vi "Convert To Child Class.vi"(11 "MetaDataObj in":refnum<class "MetaDataObj.lvclass">) -> (3 "MetaDataObj out":refnum<class "MetaDataObj.lvclass">)   [LabVIEW 2016, in "MetaDataObj.lvclass"]
uses:
  <resource>/dialog/NewProjectWizard/MetaDataObj/MetaDataObj.lvclass
  <resource>/dialog/NewProjectWizard/MetaDataObj/MetaDataObj.lvclass/MetaDataObj.ctl
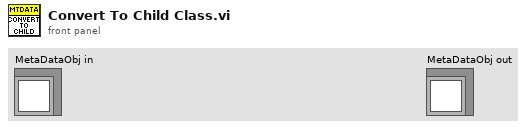
[diagram p1: front panel]
types:
  T1 = typedef "CustomVIModes.ctl" = enum16{"None", "AfterPage1", "AfterPage2WithUI", "AfterPage2NoUI"}
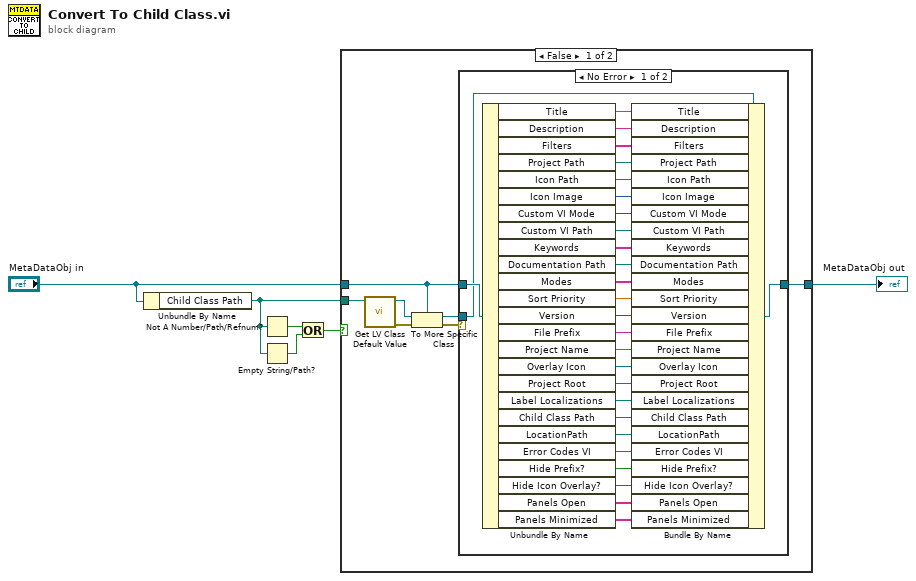
[diagram p0: block diagram]
diagram:
  n1 = Unbundle By Name("MetaDataObj in") -> ("Child Class Path"=w1:path)
  n2 = Not A Number/Path/Refnum?(number/path/refnum=w1) -> (NaN/Path/Refnum?=w6:bool)
  n3 = Empty String/Path?(string/path=w1) -> (empty?=w5:bool)
  n4 = Or(x=w6, y=w5) -> (x .or. y?=w4:bool)
  n5 = case shown="False" w4 {
    tunnel: [w8 w43] -> w3
    tunnel: "MetaDataObj in" -> [w9 w43]
    tunnel: w1 -> [w13 _]
    frame False {
      n6 = call <vilib>:"Get LV Class Default Value.vi"("class path"=w13) -> ("error out"=w7:errorcluster, "object"=w12:refnum<class>)  [unwired: 9 in]
      n7 = To More Specific Class(target class=w9, reference=w12, error in=w7) -> (specific class reference=w10:refnum<class "MetaDataObj.lvclass">, error out=w11:errorcluster)
      n8 = case shown="No Error" w11 {
        tunnel: w10 -> [w40 _]
        tunnel: w9 -> [w41 w42]
        tunnel: [w39 w42] -> w8
        frame No Error {
          n9 = Unbundle By Name(w41) -> ("Title"=w38:string, "Description"=w37:string, "Filters"=w36:string[], "Project Path"=w35:path, "Icon Path"=w34:path, "Icon Image"=w33:picture, "Custom VI Mode"=w32:T1, "Custom VI Path"=w31:path, "Keywords"=w30:string[], "Documentation Path"=w29:path, "Modes"=w28:string[], "Sort Priority"=w27:dbl, "Version"=w26:u8, "File Prefix"=w25:string, "Project Name"=w24:string, "Overlay Icon"=w23:refnum<class "Icon.lvclass">, "Project Root"=w22:path, "Label Localizations"=w21:path, "Child Class Path"=w20:path, "LocationPath"=w19:path, "Error Codes VI"=w18:path, "Hide Prefix?"=w17:bool, "Hide Icon Overlay?"=w16:bool, "Panels Open"=w15:string[], "Panels Minimized"=w14:string[])
          n10 = Bundle By Name(cluster=w40, "Title"=w38, "Description"=w37, "Filters"=w36, "Project Path"=w35, "Icon Path"=w34, "Icon Image"=w33, "Custom VI Mode"=w32, "Custom VI Path"=w31, "Keywords"=w30, "Documentation Path"=w29, "Modes"=w28, "Sort Priority"=w27, "Version"=w26, "File Prefix"=w25, "Project Name"=w24, "Overlay Icon"=w23, "Project Root"=w22, "Label Localizations"=w21, "Child Class Path"=w20, "LocationPath"=w19, "Error Codes VI"=w18, "Hide Prefix?"=w17, "Hide Icon Overlay?"=w16, "Panels Open"=w15, "Panels Minimized"=w14) -> (w39:refnum<class "MetaDataObj.lvclass">)
        }
        frame Error {
        }
      }
    }
    frame True {
    }
  }
  "MetaDataObj out" <- w3
